vi "Set Study Base.lvclass.vi"(8 "error in (no error)":errorcluster, 10 "HAL GOOP4.lvlib:Study Base.lvclass":refnum<class "Study Base.lvclass">, 11 "Study Actor in":refnum<class "Study Actor.lvclass">) -> (0 "error out":errorcluster, 3 "Study Actor out":refnum<class "Study Actor.lvclass">)   [LabVIEW 2023, in "Study Actor.lvlib" / "Study Actor.lvclass"]
uses:
  Study Actor.lvclass
  Study Base/Study Base.lvclass
  Study Actor.lvclass/Study Actor.ctl
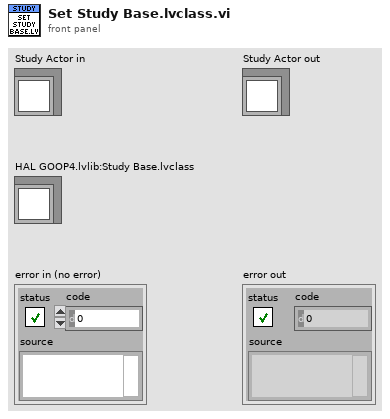
[diagram p1: front panel]
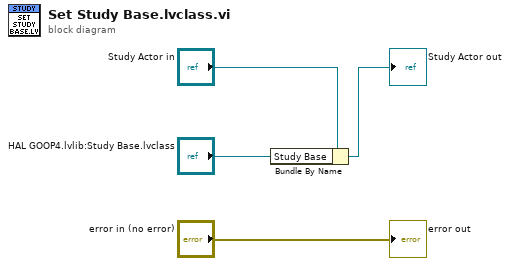
[diagram p0: block diagram]
diagram:
  n1 = Bundle By Name(cluster="Study Actor in", "Study Base"="HAL GOOP4.lvlib:Study Base.lvclass") -> (→"Study Actor out":refnum<class "Study Actor.lvclass">)
  "error out" <- "error in (no error)"
